vi "Create.vi"(5 "File Path":path, 7 "Original Name":string, 9 "MIME Type":string, 10 "Value":string, 11 "Name":string) -> (3 "FormField":refnum<class "FormField.lvclass">)   [LabVIEW 2020, in "HTTP Utils.lvlib" / "FormField.lvclass"]
uses:
  FormField.lvclass
  FormField.lvclass/FormField.ctl
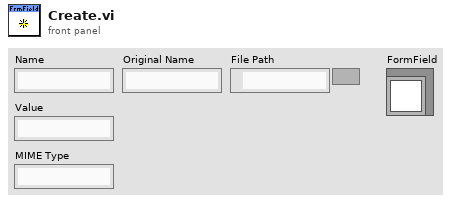
[diagram p1: front panel]
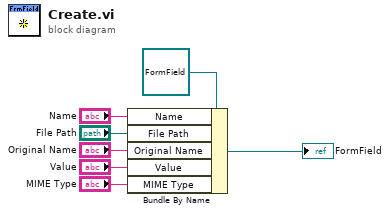
[diagram p0: block diagram]
diagram:
  n1 = Bundle By Name(cluster=refnum<class "FormField.lvclass"> refnum ("HTTP Utils.lvlib:FormField"), "Name"="Name", "File Path"="File Path", "Original Name"="Original Name", "Value"="Value", "MIME Type"="MIME Type") -> (→"FormField":refnum<class "FormField.lvclass">)
